vi "Voltage_overflow_checker.vi"(2 "Voltages":dbl[][](array[numeric])) -> (0 "Over/Under string":string)   [LabVIEW 2013]
uses:
  Globals/Meas_global.vi
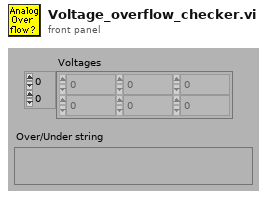
[diagram p1: front panel]
types:
  T1 = typedef "Ch_and_Spans.ctl" = cluster{"high limit (10V)":sgl, "low limit (-10V)":sgl, "Ch No":i16, "Var name":string, "Use Latest Calib":bool}
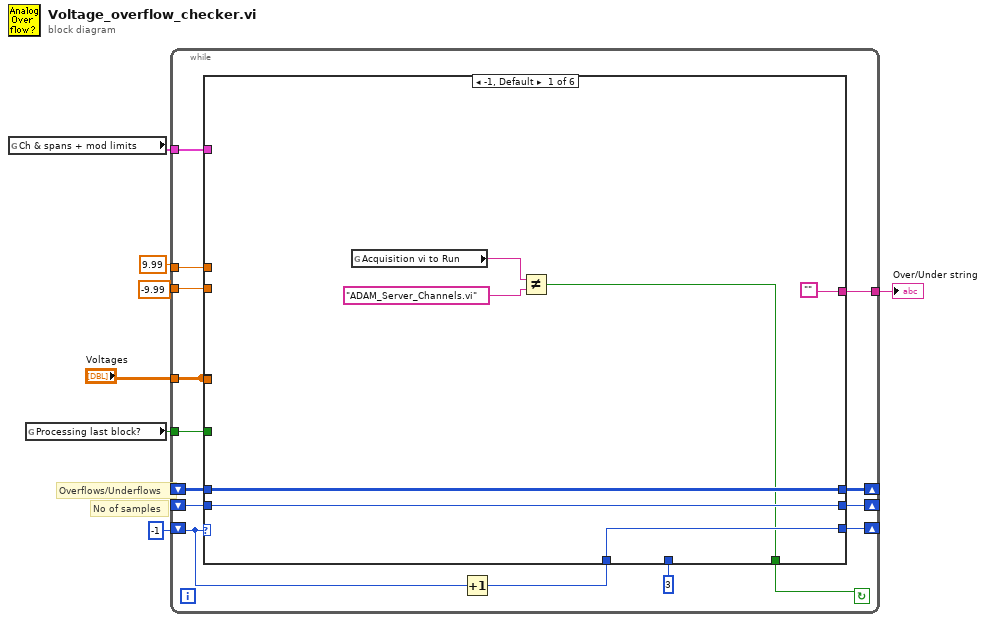
[diagram p0: block diagram]
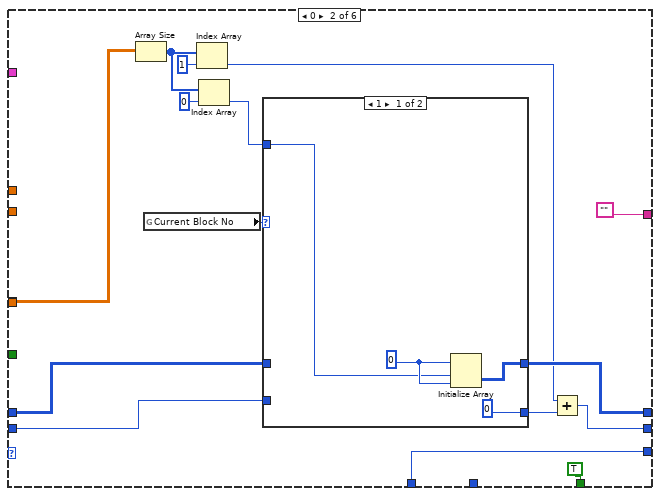
[diagram p2: hidden frame]
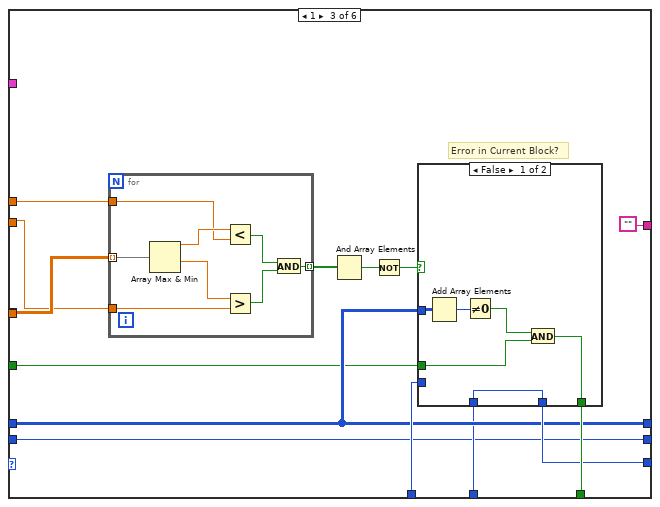
[diagram p4: hidden frame]
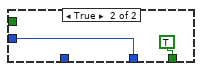
[diagram p5: hidden frame]
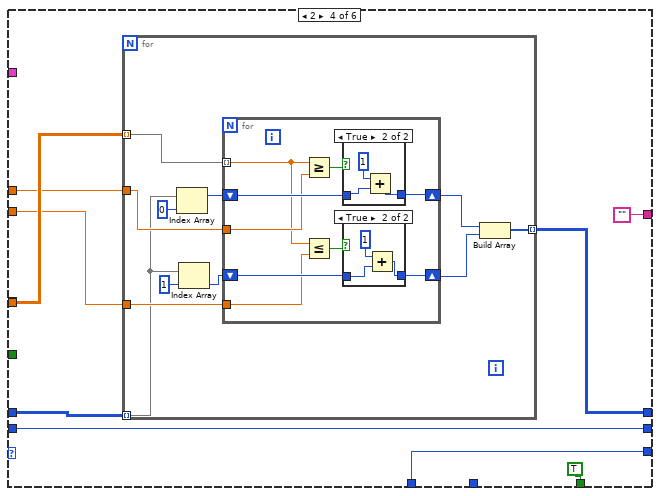
[diagram p6: hidden frame]
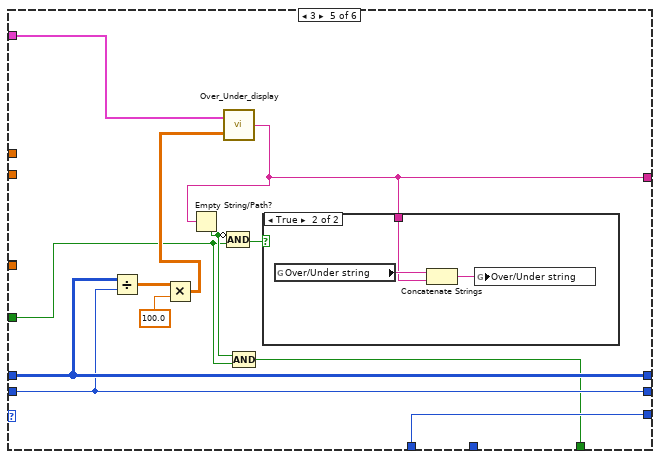
[diagram p9: hidden frame]
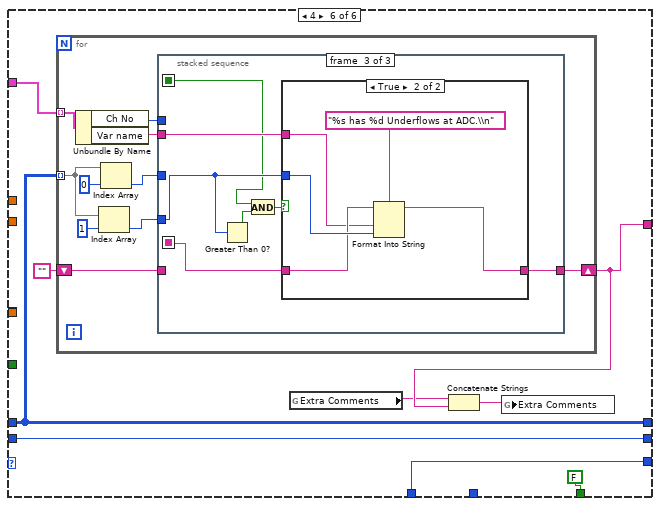
[diagram p11: hidden frame]
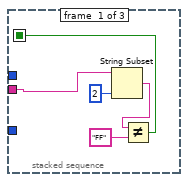
[diagram p12: hidden frame]
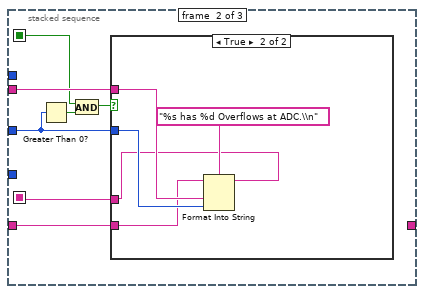
[diagram p13: hidden frame]
diagram:
  # "No of samples"
  # "Overflows/Underflows"
  n1 = global read "Meas_global.vi" "Ch & spans + mod limits"() -> (w3:T1[])
  n2 = global read "Meas_global.vi" "Processing last block?"() -> (w5:bool)
  n3 = while {
    tunnel: [w8] -> w4
    tunnel: w5 -> [w10]
    shift-left: _ -> [w14]
    shift-right: [w11] -> _
    shift-left: _ -> [w13]
    shift-right: [w12] -> _
    tunnel: "Voltages" -> [w15]
    shift-left: -1 -> [w18]
    shift-right: [w16] -> _
    tunnel: -9.99 -> [w20]
    tunnel: 9.99 -> [w21]
    tunnel: w3 -> [w22]
    stop <- w19 continue-if-true
    n4 = Increment(x=w18) -> (x+1=w17:i32)
    n5 = case shown="-1, Default" w18 {
      tunnel: w22 -> [_ _ _ _ w128 w136]
      tunnel: w21 -> [_ _ w63 w87 _ _]
      tunnel: w20 -> [_ _ w62 w88 _ _]
      tunnel: w15 -> [_ w36 w64 _ _ _]
      tunnel: [w23 TRUE w59 TRUE w118 FALSE] -> w19
      tunnel: w17 -> [w26 w39 w57 w85 w129 w141]
      tunnel: [w26 w39 w58 w85 w129 w141] -> w16
      tunnel: w15 -> [_ _ _ w89 _ _]
      tunnel: w14 -> [w27 w42 w53 w81 w126 w140]
      tunnel: w13 -> [w28 w40 w56 w82 w127 w137]
      tunnel: [w28 w43 w56 w86 w127 w137] -> w12
      tunnel: [w27 w33 w53 w81 w126 w140] -> w11
      tunnel: w10 -> [_ _ w51 _ w119 _]
      tunnel: 3 -> [_ _ w55 _ _ _]
      tunnel: ["" "" "" "" w121 w134] -> w8
      frame -1, Default {
        n6 = global read "Meas_global.vi" "Acquisition vi to Run"() -> (w24:string)
        n7 = Not Equal?(x=w24, y="ADAM_Server_Channels.vi" ("Acquisition vi to Run")) -> (x != y?=w23:bool)
      }
      frame 0 {
        n8 = Array Size(array=w36) -> (size(s)=w31:i32[])
        n9 = global read "Meas_global.vi" "Current Block No"() -> (w44:i32)
        n10 = Index Array(array=w31, index=1 ("Index")) -> (element=w35:i32)
        n11 = Index Array(array=w31, index=0 ("Index")) -> (element=w30:i32)
        n12 = case shown="1" w44 {
          tunnel: [w48 w50] -> w43
          tunnel: w40 -> [_ w50]
          tunnel: w42 -> [_ w49]
          tunnel: [0 w49] -> w34
          tunnel: w30 -> [w45 _]
          frame 1 {
            w46 = 0
            n13 = Initialize Array(w46, w45, w46) -> (w48:i32[][])
          }
          frame 2, Default {
          }
        }
        n14 = Add(x=w35, y=w34) -> (x+y=w33:i32)
      }
      frame 1 {
        # "Error in Current Block?"
        n15 = for {
          tunnel: w64 -> [w80] mode=indexing
          tunnel: w63 -> [w78]
          tunnel: w62 -> [w76]
          tunnel: [w73] -> w61 mode=indexing
          n16 = Array Max & Min(array=w80) -> (max value=w79:dbl, min value=w77:dbl)  [unwired: 2 out]
          n17 = Less?(x=w79, y=w78) -> (x < y?=w74:bool)
          n18 = Greater?(x=w77, y=w76) -> (0:w75:bool)
          n19 = And(x=w74, y=w75) -> (x .and. y?=w73:bool)
        }
        n20 = And Array Elements(Boolean array=w61) -> (logical AND=w60:bool)
        n21 = Not(x=w60) -> (.not. x?=w52:bool)
        n22 = case shown="False" w52 {
          tunnel: [w66 TRUE] -> w59
          tunnel: [w65 w71] -> w58
          tunnel: w57 -> [_ w71]
          tunnel: w56 -> [w70 _]
          tunnel: w55 -> [w65 _]
          tunnel: w51 -> [w67 _]
          frame False {
            n23 = Add Array Elements(numeric array=w70) -> (sum=w69:i32)
            n24 = Not Equal To 0?(x=w69) -> (x != 0?=w68:bool)
            n25 = And(x=w68, y=w67) -> (x .and. y?=w66:bool)
          }
          frame True {
          }
        }
      }
      frame 2 {
        n26 = for {
          tunnel: w89 -> [w98] mode=indexing
          tunnel: w88 -> [w100]
          tunnel: w87 -> [w99]
          tunnel: [w96] -> w86 mode=indexing
          tunnel: w82 -> [w92] mode=indexing
          n27 = Index Array(array=w92, index=0 ("Index")) -> (element=w90:i32)
          n28 = Index Array(array=w92, index=1 ("Index")) -> (element=w91:i32)
          n29 = for {
            shift-right: [w104] -> w95
            shift-left: w91 -> [w105]
            shift-right: [w107] -> w97
            shift-left: w90 -> [w108]
            tunnel: w98 -> [w101] mode=indexing
            tunnel: w100 -> [w103]
            tunnel: w99 -> [w102]
            n30 = Greater Or Equal?(x=w101, y=w102) -> (x >= y?=w109:bool)
            n31 = Less Or Equal?(x=w101, y=w103) -> (x <= y?=w106:bool)
            n32 = case shown="True" w109 {
              tunnel: [w114 w116] -> w107
              tunnel: w108 -> [w114 w117]
              frame False {
              }
              frame True {
                n33 = Add(x=1, y=w117) -> (x+y=w116:i32)
              }
            }
            n34 = case shown="True" w106 {
              tunnel: w105 -> [w110 w112]
              tunnel: [w110 w111] -> w104
              frame False {
              }
              frame True {
                n35 = Add(x=1, y=w112) -> (x+y=w111:i32)
              }
            }
          }
          n36 = Build Array(w97, w95) -> (w96:i32[])
        }
      }
      frame 3 {
        n37 = Divide(x=w127, y=w126) -> (x/y=w125:dbl[][])
        n38 = Multiply(x=w125, y=100.0) -> (x*y=w123:dbl[][])
        n39 = call "Over_Under_display.vi"("Overflow array"=w123, "Ch & spans"=w128) -> ("Over/Under string"=w121:string)
        n40 = Empty String/Path?(string/path=w121) -> (empty?=w120:bool)
        n41 = Compound Arithmetic op=AND(invert w120, w119) -> (w122:bool)
        n42 = Compound Arithmetic op=AND(w120, w119) -> (w118:bool)
        n43 = case shown="True" w122 {
          tunnel: w121 -> [_ w130]
          frame False {
          }
          frame True {
            n44 = global read "Meas_global.vi" "Over/Under string"() -> (w132:string)
            n45 = Concatenate Strings(w132, w130) -> (w131:string)
            n46 = global write "Meas_global.vi" "Over/Under string"(w131) -> ()
          }
        }
      }
      frame 4 {
        n47 = for {
          tunnel: w136 -> [w151] mode=indexing
          tunnel: w137 -> [w150] mode=indexing
          shift-right: [w142] -> w134
          shift-left: "" -> [w143]
          n48 = Unbundle By Name(w151) -> ("Ch No"=w149:i16, "Var name"=w148:string)
          n49 = Index Array(array=w150, index=1) -> (element=w144:i32)
          n50 = Index Array(array=w150, index=0) -> (element=w145:i32)
          n51 = stacked-sequence {
            seq-local: [_ w161 _] -> [_ _ w176]
            seq-local: [w152 _ _] -> [_ w158 w170]
            tunnel: w144 -> [_ _ w174]
            tunnel: w145 -> [_ w160 _]
            tunnel: w148 -> [w153 w163 w173]
            tunnel: w149 -> [_ _ _]
            tunnel: w143 -> [_ w162 _]
            tunnel: [_ _ w175] -> w142
            frame #0 {
              n52 = String Subset(string=w153, length (rest)=2 ("length (rest)")) -> (substring=w155:string)  [unwired: 1 out]
              n53 = Not Equal?(x=w155, y="FF") -> (x != y?=w152:bool)
            }
            frame #1 {
              n54 = Greater Than 0?(x=w160) -> (x > 0?=w159:bool)
              n55 = And(x=w158, y=w159) -> (x .and. y?=w157:bool)
              n56 = case shown="True" w157 {
                tunnel: w160 -> [_ w167]
                tunnel: w163 -> [_ w168]
                tunnel: w162 -> [w164 w166]
                tunnel: [w164 w165] -> w161
                frame False {
                }
                frame True {
                  n57 = Format Into String(format string="%s has %d Overflows at ADC.\\n" ("Format String"), initial string=w166, w168, w167) -> (resulting string=w165:string)  [unwired: 1 in, 1 out]
                }
              }
            }
            frame #2 {
              n58 = Greater Than 0?(x=w174) -> (x > 0?=w172:bool)
              n59 = And(x=w170, y=w172) -> (x .and. y?=w171:bool)
              n60 = case shown="True" w171 {
                tunnel: w174 -> [_ w182]
                tunnel: w173 -> [_ w178]
                tunnel: w176 -> [w177 w181]
                tunnel: [w177 w180] -> w175
                frame False {
                }
                frame True {
                  n61 = Format Into String(format string="%s has %d Underflows at ADC.\\n" ("Format String"), initial string=w181, w178, w182) -> (resulting string=w180:string)  [unwired: 1 in, 1 out]
                }
              }
            }
          }
        }
        n62 = global read "Meas_global.vi" "Extra Comments"() -> (w133:string)
        n63 = Concatenate Strings(w133, w134) -> (w138:string)
        n64 = global write "Meas_global.vi" "Extra Comments"(w138) -> ()
      }
    }
  }
  "Over/Under string" <- w4
